vi "Exit Open Instruments.vi"(8 "error in (no error)":errorcluster, 10 "Instrument Names":string[](array[string]), 11 "Master":refnum<queue>) -> (0 "error out":errorcluster)   [LabVIEW 2013]
uses:
  MeasurementControl Message Queue Folder/Message Cluster.ctl
  MeasurementControl Message Queue Folder/MeasurementControl Message Queue.lvlib
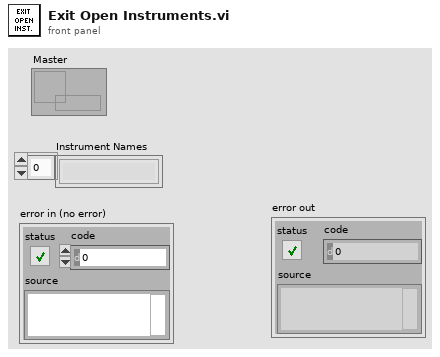
[diagram p1: front panel]
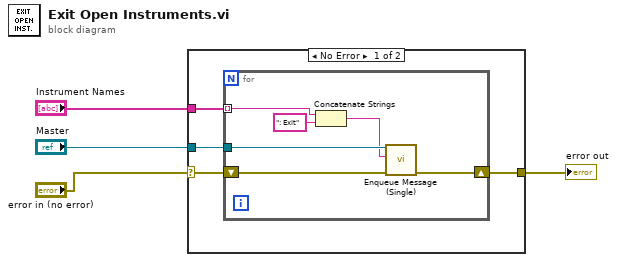
[diagram p0: block diagram]
diagram:
  n1 = case shown="No Error" "error in (no error)" {
    selector: "error in (no error)" -> [w5 w15]
    tunnel: "Instrument Names" -> [w8 _]
    tunnel: "Master" -> [w7 _]
    tunnel: [w6 w15] -> w1
    frame No Error {
      n2 = for {
        tunnel: w8 -> [w13] mode=indexing
        tunnel: w7 -> [w12]
        shift-right: [w10] -> w6
        shift-left: w5 -> [w9]
        n3 = Concatenate Strings(w13, ": Exit" ("string")) -> (w11:string)
        n4 = call "Enqueue Message (Single).vi"("error in (no error)"=w9, "Message"=w11, "Message Queue"=w12) -> ("error out"=w10:errorcluster)  [unwired: 7 in, 1 out]
      }
    }
    frame Error {
    }
  }
  "error out" <- w1
